vi "FXP NIPLL_VCO.vi"(9 "nominal freq [U16.0]":fxp<+,16,0>, 10 "Kv [U16.0]":fxp<+,16,0>, 11 "v [I48.17]":fxp<+/-,48,17>) -> (0 "f":fxp<+/-,32,0> format="%.32g", 1 "z [I32.1]":fxp<+/-,32,1>, 2 "sin(z) [I16.2]":fxp<+/-,16,2> format="%.15g", 3 "cos(z) [I16.2]":fxp<+/-,16,2> format="%.15g")   [LabVIEW 2016]
uses:
  <vilib>/rvi/FXPMathLib/FxpConvert/subVIs/nifxpmath_Convert_SimConfig.ctl
  <vilib>/fxp/LVFixedPointQuantizationPolicyTypeDef.ctl
  <vilib>/fxp/LVFixedPointOverflowPolicyTypeDef.ctl
  <vilib>/rvi/FXPMathLib/basic elements/FxpIntAccumulator/subVIs/nifxpmath_IntAccumulator_SimConfig.ctl
  <vilib>/rvi/FXPMathLib/FxpSinAndCos/subVIs/nifxpmath_SinAndCos_SimConfig.ctl
  <vilib>/rvi/FXPMathLib/FxpConvert/simVIs/DllFxpConvertTemp_sub.vi
  <vilib>/rvi/FXPMathLib/basic elements/FxpIntAccumulator/simVIs/DllFxpIntAccumulator_sub.vi
  <vilib>/rvi/FXPMathLib/FxpSinAndCos/simVIs/DllFxpSinAndCosTemp_sub.vi
  <vilib>/rvi/FXPMathLib/FxpConvert/XNode/nifxpmath_Convert.xnode
  <vilib>/rvi/FXPMathLib/FxpMul/XNode/nifxpmath_Multiplier.xnode
  <vilib>/rvi/FXPMathLib/FxpAdd/XNode/nifxpmath_Add.xnode
  <vilib>/rvi/FXPMathLib/basic elements/FxpIntAccumulator/XNode/nifxpmath_IntAccumulator.xnode
  <vilib>/rvi/FXPMathLib/FxpSinAndCos/XNode/nifxpmath_SinAndCos.xnode
  <vilib>/rvi/FXPMathLib/sim/FxpSim.dll
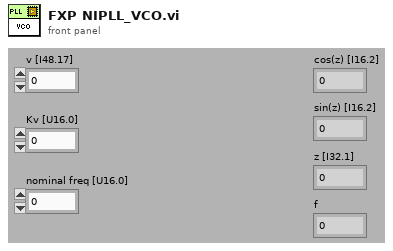
[diagram p1: front panel]
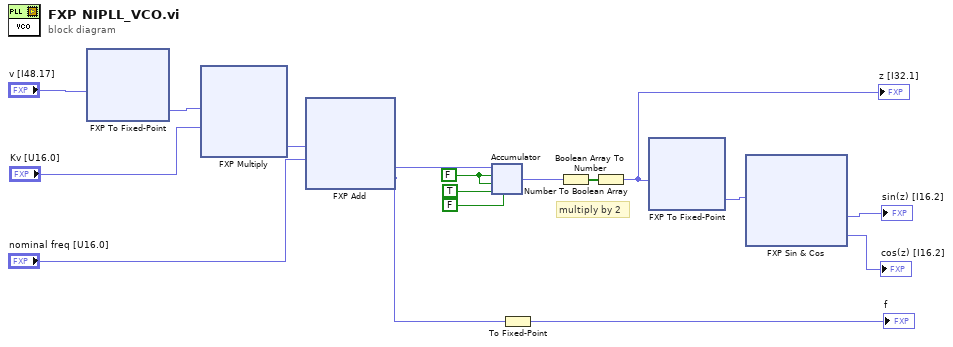
[diagram p0: block diagram]
diagram:
  w11 = FALSE ("is sub")
  # "multiply by 2"
  n1 = xnode "FXP To Fixed-Point"("x"="v [I48.17]") -> ("y"=w4:fxp<+/-,32,17>)
  n2 = xnode "FXP Multiply"("x"=w4, "y"="Kv [U16.0]") -> ("x*y"=w8:fxp<+/-,32,0>)
  n3 = xnode "FXP Add"("x"=w8, "y"="nominal freq [U16.0]") -> ("x+y"=w6:fxp<+/-,32,0>)
  n4 = xnode "Accumulator"("x"=w6, "load (F)"=w11, "is sub? (F)"=w11, "enable (T)"=TRUE ("enable"), "carry-in/inverted borrow-in (F)"=FALSE ("cin/nbin")) -> ("s"=w3:fxp<+/-,32,0>)  [unwired: 1 out]
  n5 = To Fixed-Point(number=w6) -> (fixed-point=→"f":fxp<+/-,32,0>)  [unwired: 1 in]
  n6 = Number To Boolean Array(number=w3) -> (Boolean array=w7:bool[])
  n7 = Boolean Array To Number(Boolean array=w7) -> (number=w2:fxp<+/-,32,1>)
  "z [I32.1]" <- w2
  n8 = xnode "FXP To Fixed-Point"("x"=w2) -> ("y"=w1:fxp<+/-,16,1>)
  n9 = xnode "FXP Sin & Cos"("x (pi)"=w1) -> ("sin(x)"=→"sin(z) [I16.2]":fxp<+/-,16,2>, "cos(x)"=→"cos(z) [I16.2]":fxp<+/-,16,2>)
